vi "Set Start Parameter.vi"(8 "error in (no error)":errorcluster, 10 "Start Parameter":T1={"Windows Titel"="", "Start WorkDir"=path "", "Camera ConfigDir"=path "", "Camera"="", "OverlayColor"=13816530, "TimeInFilename"=FALSE, "TimestampFormat"="%H.%M.%S%3u", "ShotIdInFilename"=FALSE, "CamInFilename"=FALSE, "FrameNrInFilename"=FALSE}, 11 "HIJ Vision Launcher in":refnum<class "HIJ Vision Launcher.lvclass">) -> (0 "error out":errorcluster, 3 "HIJ Vision Launcher out":refnum<class "HIJ Vision Launcher.lvclass">)   [LabVIEW 2020, in "HIJ Vision Launcher.lvlib" / "HIJ Vision Launcher.lvclass"]
uses:
  HIJ Vision Launcher.lvclass
  C:/Users/AlexK/work/LabVIEW Programme/POLARIS CAM Log Abw und E/Submodules/Viewable Actor/ViewableActor/ViewableActor.lvclass
  Start Parameter.ctl
  <vilib>/userdefined/High Color/IMAQdx.ctl
  Application Base Actors/HIJ Vision Camera App/HIJ Vision Camera App/HIJ Vision Camera App.lvclass
  C:/Users/AlexK/work/LabVIEW Programme/POLARIS CAM Log Abw und E/Submodules/HIJ Vision/Application Base Actors/HIJ Vision Application/HIJ Vision Application/HIJ Vision Application.lvclass
  Viewable Actor/ViewableActor/ViewableActor.lvclass/ViewableActor.ctl
  HIJ Vision Launcher.lvclass/HIJ Vision Launcher.ctl
  Application Base Actors/HIJ Vision Camera App/HIJ Vision Camera App/HIJ Vision Camera App.lvclass/HIJ Vision Camera App.ctl
  Viewable Actor/ViewableActor/Read Config URL.vi
  Read Cmd Parameters.vi
  Application Base Actors/HIJ Vision Camera App/HIJ Vision Camera App/Write OverlayColor.vi
  Application Base Actors/HIJ Vision Camera App/HIJ Vision Camera App/Write SaveTimestamp.vi
  Application Base Actors/HIJ Vision Camera App/HIJ Vision Camera App/Write TimestampFormat.vi
  Application Base Actors/HIJ Vision Camera App/HIJ Vision Camera App/Write ShotIdInFileName.vi
  Application Base Actors/HIJ Vision Camera App/HIJ Vision Camera App/Write Save Source in Filename.vi
  Application Base Actors/HIJ Vision Camera App/HIJ Vision Camera App/Write FrameNrInFilename.vi
  Viewable Actor/ViewableActor/Write Config URL.vi
  Application Base Actors/HIJ Vision Camera App/HIJ Vision Camera App/Write CMD Line .vi
  Application Base Actors/HIJ Vision Camera App/HIJ Vision Camera App/Write Camera Name.vi
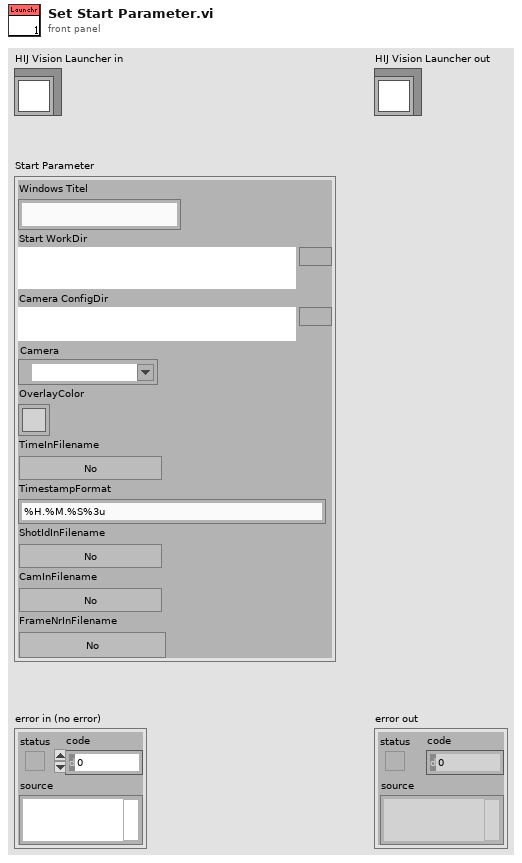
[diagram p1: front panel]
types:
  T1 = typedef "HIJ Vision Launcher.lvlib/HIJ Vision Launcher.lvclass/Start Parameter.ctl" = cluster{"Windows Titel":string, "Start WorkDir":path, "Camera ConfigDir":path, "Camera":T2, "OverlayColor":u32, "TimeInFilename":bool, "TimestampFormat":string, "ShotIdInFilename":bool, "CamInFilename":bool, "FrameNrInFilename":bool}
  T2 = typedef "IMAQdx.ctl" = refnum<k21>
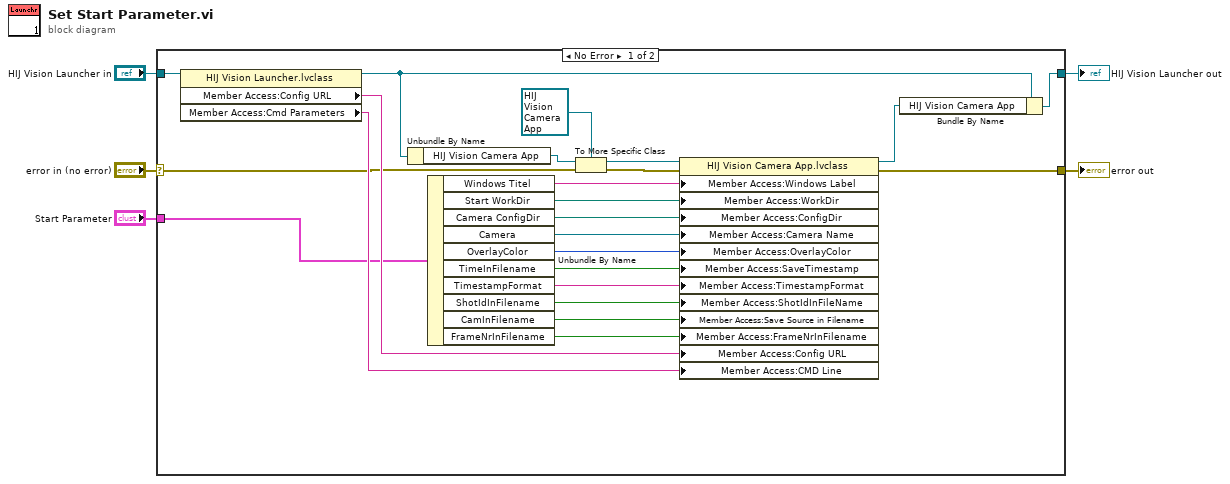
[diagram p0: block diagram]
diagram:
  n1 = case shown="No Error" "error in (no error)" {
    selector: "error in (no error)" -> [w15 w30]
    tunnel: [w18 w30] -> w4
    tunnel: [w26 w29] -> w2
    tunnel: "HIJ Vision Launcher in" -> [w25 w29]
    tunnel: "Start Parameter" -> [w23 _]
    frame No Error {
      n2 = property class="HIJ Vision Launcher.lvclass"(reference=w25) -> (reference out=w12:refnum<class "HIJ Vision Launcher.lvclass">, "Member Access:Config URL"=w28:string, "Member Access:Cmd Parameters"=w27:string)  [unwired: 1 in, 1 out]
      n3 = Unbundle By Name(w12) -> ("HIJ Vision Camera App"=w16:refnum<class "ViewableActor.lvclass">)
      n4 = Unbundle By Name(w23) -> ("Windows Titel"=w22:string, "Start WorkDir"=w21:path, "Camera ConfigDir"=w20:path, "Camera"=w19:T2, "OverlayColor"=w11:u32, "TimeInFilename"=w10:bool, "TimestampFormat"=w9:string, "ShotIdInFilename"=w8:bool, "CamInFilename"=w7:bool, "FrameNrInFilename"=w6:bool)
      n5 = To More Specific Class(target class=refnum<class "HIJ Vision Camera App.lvclass"> refnum ("HIJ Vision Camera App.lvlib:HIJ Vision Camera App.lvclass"), reference=w16, error in=w15) -> (specific class reference=w17:refnum<class "HIJ Vision Camera App.lvclass">, error out=w14:errorcluster)
      n6 = property class="HIJ Vision Camera App.lvclass"(reference=w17, error in=w14, "Member Access:Windows Label"=w22, "Member Access:WorkDir"=w21, "Member Access:ConfigDir"=w20, "Member Access:Camera Name"=w19, "Member Access:OverlayColor"=w11, "Member Access:SaveTimestamp"=w10, "Member Access:TimestampFormat"=w9, "Member Access:ShotIdInFileName"=w8, "Member Access:Save Source in Filename"=w7, "Member Access:FrameNrInFilename"=w6, "Member Access:Config URL"=w28, "Member Access:CMD Line "=w27) -> (reference out=w24:refnum<class "HIJ Vision Camera App.lvclass">, error out=w18:errorcluster)
      n7 = Bundle By Name(cluster=w12, "HIJ Vision Camera App"=w24) -> (w26:refnum<class "HIJ Vision Launcher.lvclass">)
    }
    frame Error {
    }
  }
  "error out" <- w4
  "HIJ Vision Launcher out" <- w2
